vi "Installer.vi"() -> ()   [LabVIEW 2019, in "ByteLVDevEnv.lvlib"]
doc: "VIP Package Installer.\nTakes a txt file with libraries version you want to install and automatically imports them into VIPM and installs them.\nThe txt needs to be formatted this way:\nLibName == 1.1.1.1\nor\n0.0.0.0 > LibName <= 1.1.1.1\nOne library version for line."
uses:
  ByteLVDevEnv.lvlib
  TypeDefs/LibraryVersions.ctl
  TypeDefs/AllLibraries.ctl
  <vilib>/regexp/Match Regular Expression.xnode
  <vilib>/JKI/VIPM API/VIPM API_vipm_api.lvlib
panel:
  in  "Select LabVIEV Version":u16(ring) items=["19.0"]
  out "Status":string
  in  "Exit":bool
  in  "Restart":bool
  out "LOADING":string
  out "Packets file errors":string[](array[string])
  in  "Local VIP Folder":path
  out "VIP files found in local folder":string
  out "Install log":string[](array[string])
  in  "Start":bool
  in  "Packets File Path":path
  # "Development Environment"
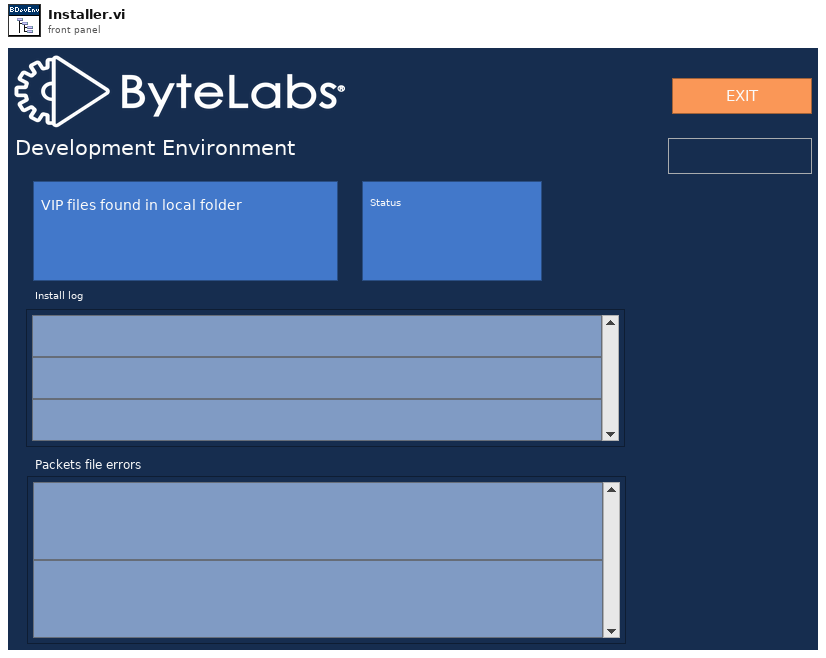
[diagram p1: front panel]
types:
  T1 = typedef "ByteLVDevEnv.lvlib/AllLibraries.ctl" = cluster{"Package Name":string, "Version":string, "Installed":bool, "Path":path}
  T2 = typedef "ByteLVDevEnv.lvlib/LibraryVersions.ctl" = cluster{"Name":string, "Version 1 ":string, "Version 2":string, "Sign 1":string, "Sign 2":string, "Function":string, "V. Install":string}
  T3 = cluster{"LOADING":refnum<vi>, "Local VIP Folder":refnum<vi>, "Packets File Path ":refnum<vi>, "Start":refnum<vi>, "Install log":refnum<vi>, "VIP files found in local folder":refnum<vi>, "Packets file errors":refnum<vi>, "Restart":refnum<vi>, "Exit":refnum<vi>, "Status":refnum<vi>, "Select LabVIEV Version":refnum<vi>}
  T4 = cluster{"Status":string, "Versions":T2[], "All Packages":T1[], "LabView V.":string, "LocalVip":T1[], "Log":string[], "Packets errors":string[]}
  T5 = enum8{"Enabled", "Disabled", "Disabled and Grayed Out"}
  T6 = enum16{"open", "replace", "create", "open or create", "replace or create", "replace or create with confirmation"}
  T7 = cluster{"Packets File Path ":path, "Local VIP Folder":path, "Select LabVIEV Version":u16}
  T8 = typedef "VIPM API_vipm_api.lvlib/LabVIEW Target Info Cluster_vipm_api.ctl" = cluster{"Version":string, "Connection Tested":bool, "Disabled":bool}
  T9 = typedef "LVStringsAndValuesArrayTypeDef_U16.ctl" = cluster{"String":string, "Value":u16}[]
  T10 = typedef "VIPM API_vipm_api.lvlib/Library Contents Cluster_vipm_api.ctl" = cluster{"Package Name":string, "Version":string, "Display Name":string, "Repository Name":string, "Company Name":string, "License Type":string, "Installed":bool, "Deprecated":bool, "Dependency or Conflict Problem":bool, "Downloaded":bool}
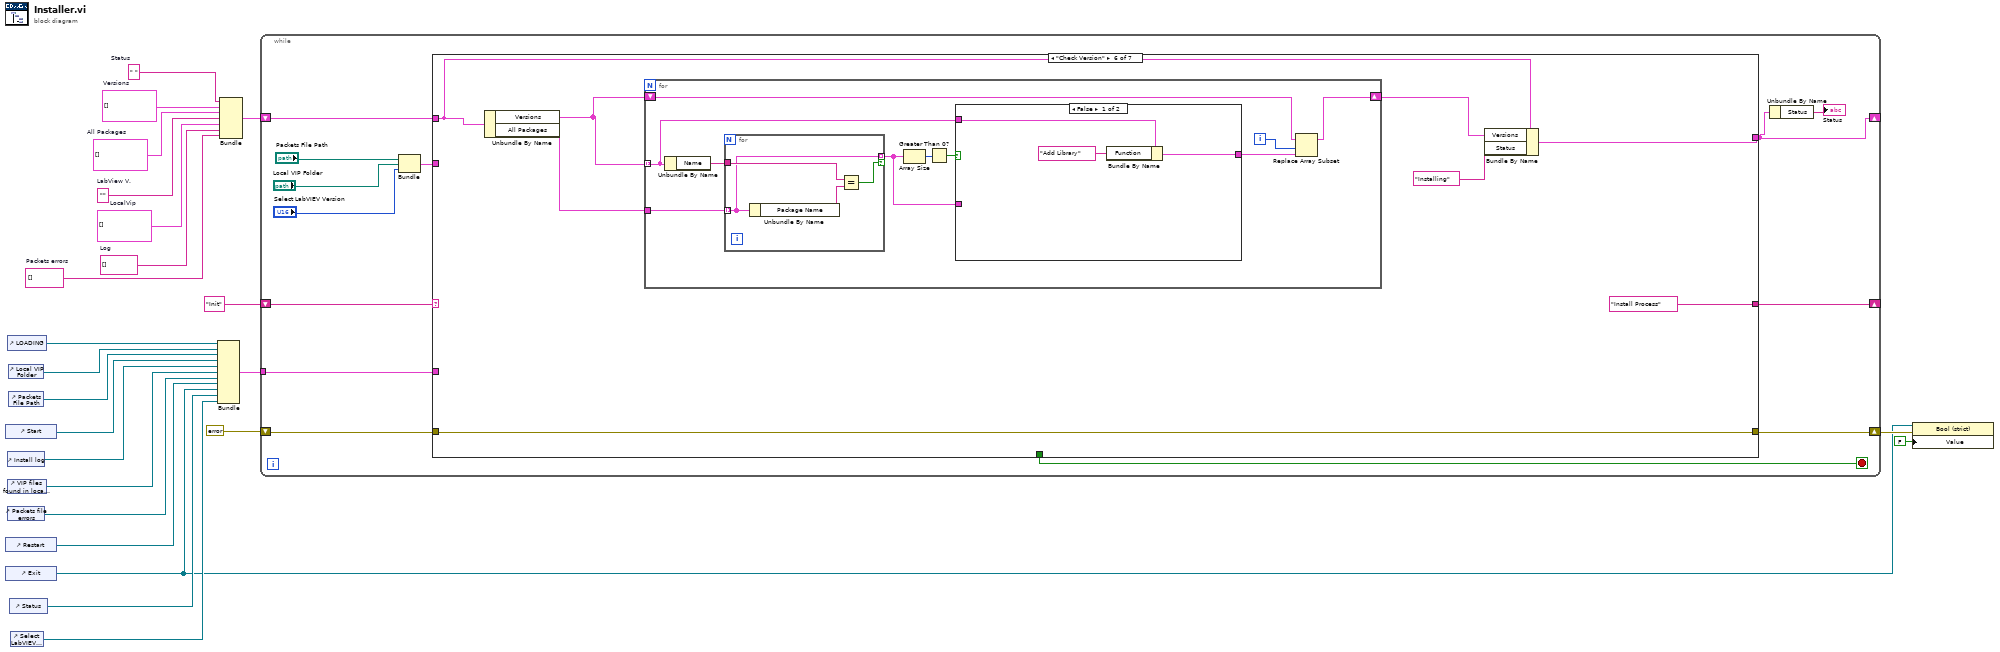
[diagram p0: block diagram]
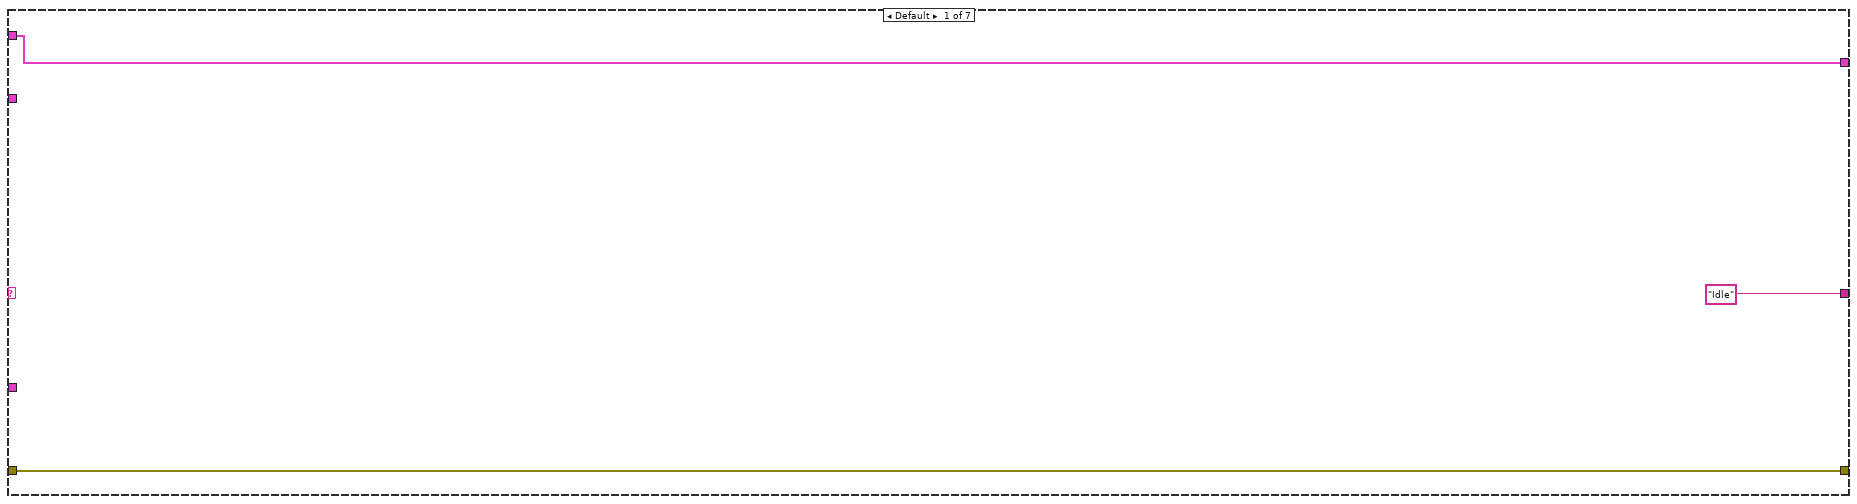
[diagram p2: hidden frame]
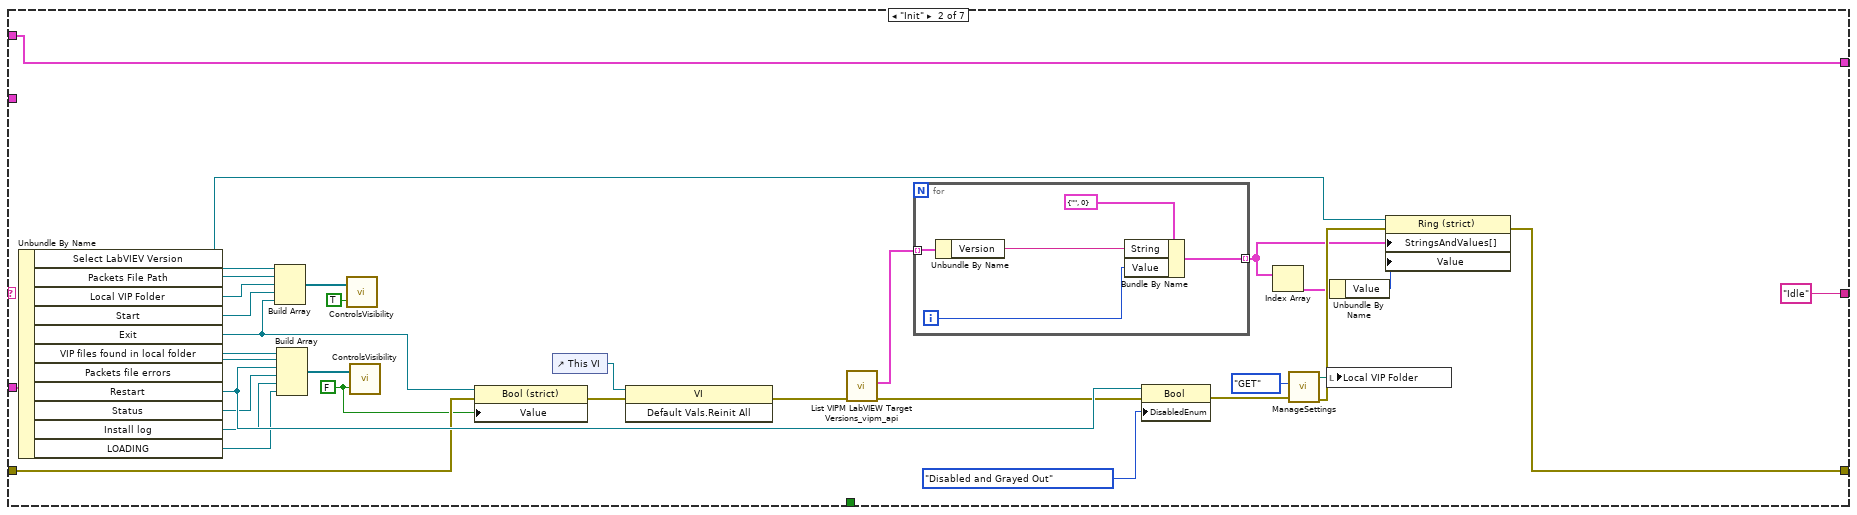
[diagram p3: hidden frame]
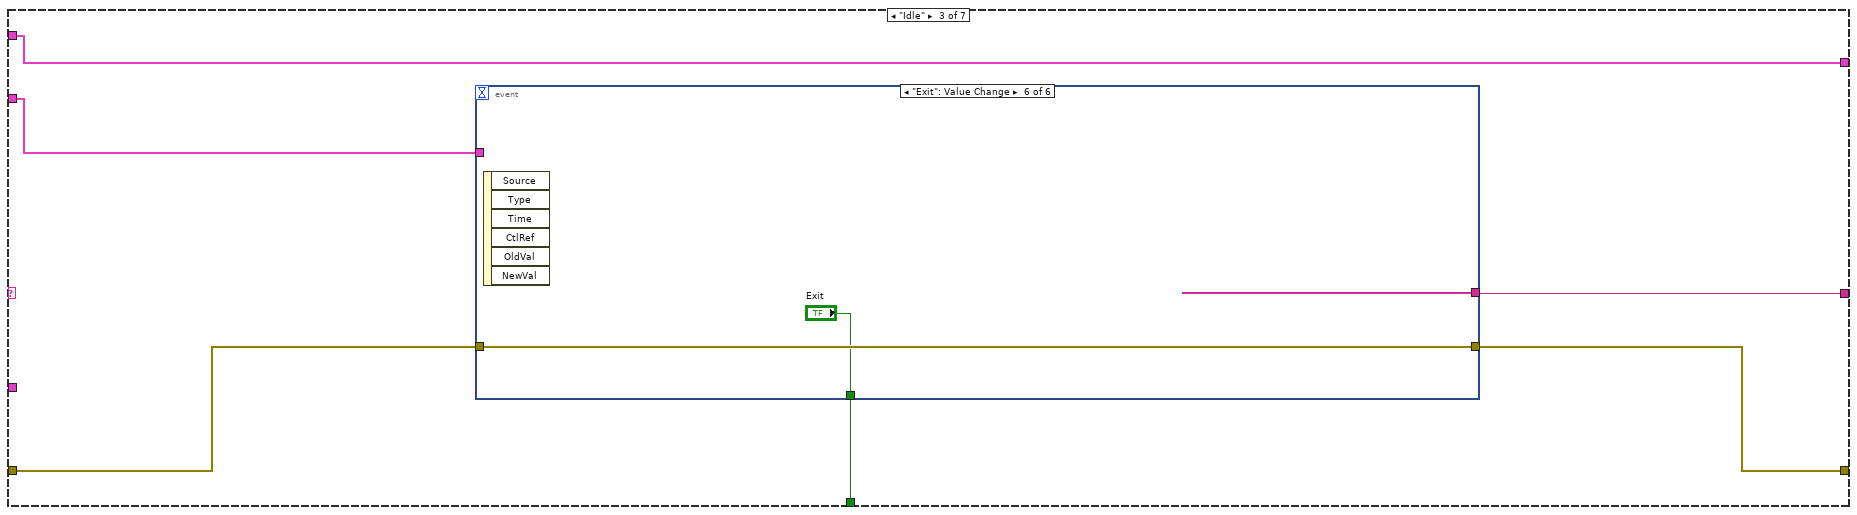
[diagram p4: hidden frame]
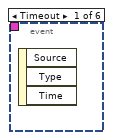
[diagram p5: hidden frame]
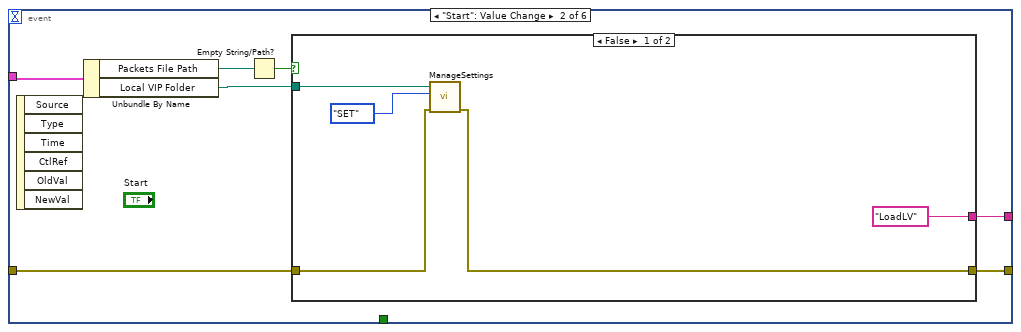
[diagram p6: hidden frame]
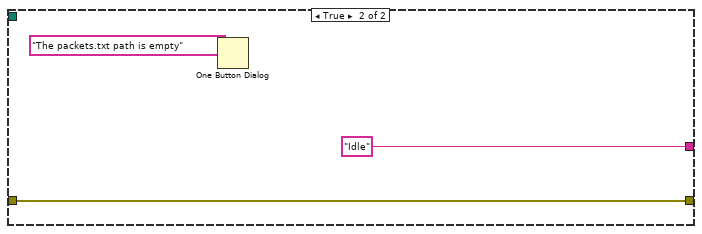
[diagram p7: hidden frame]
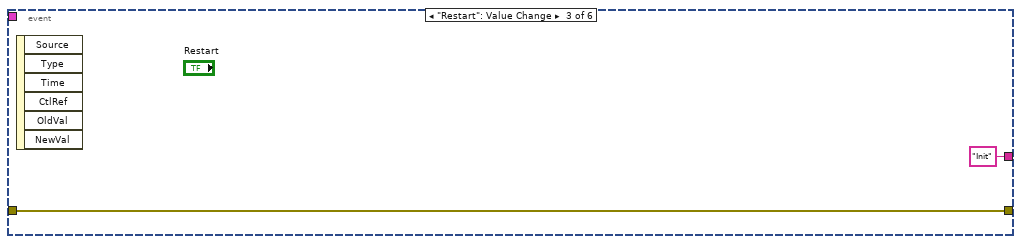
[diagram p8: hidden frame]
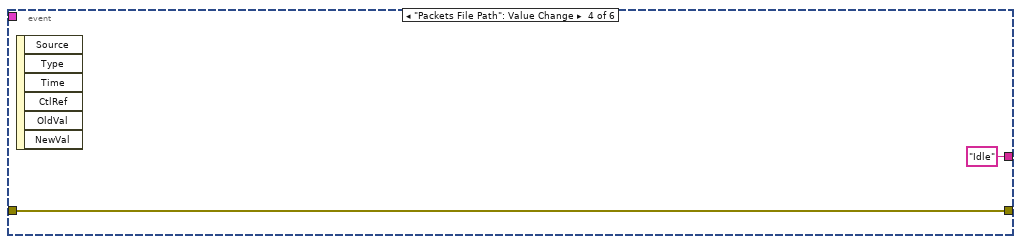
[diagram p9: hidden frame]
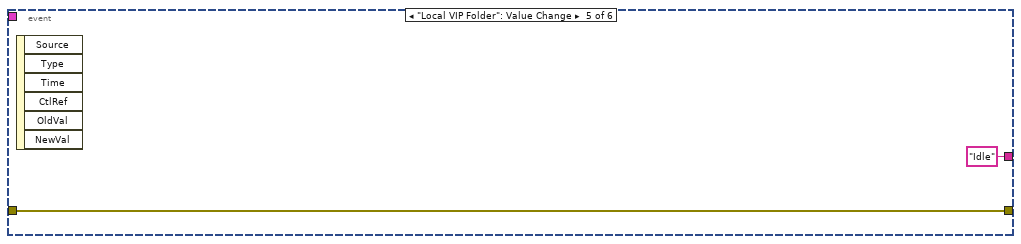
[diagram p10: hidden frame]
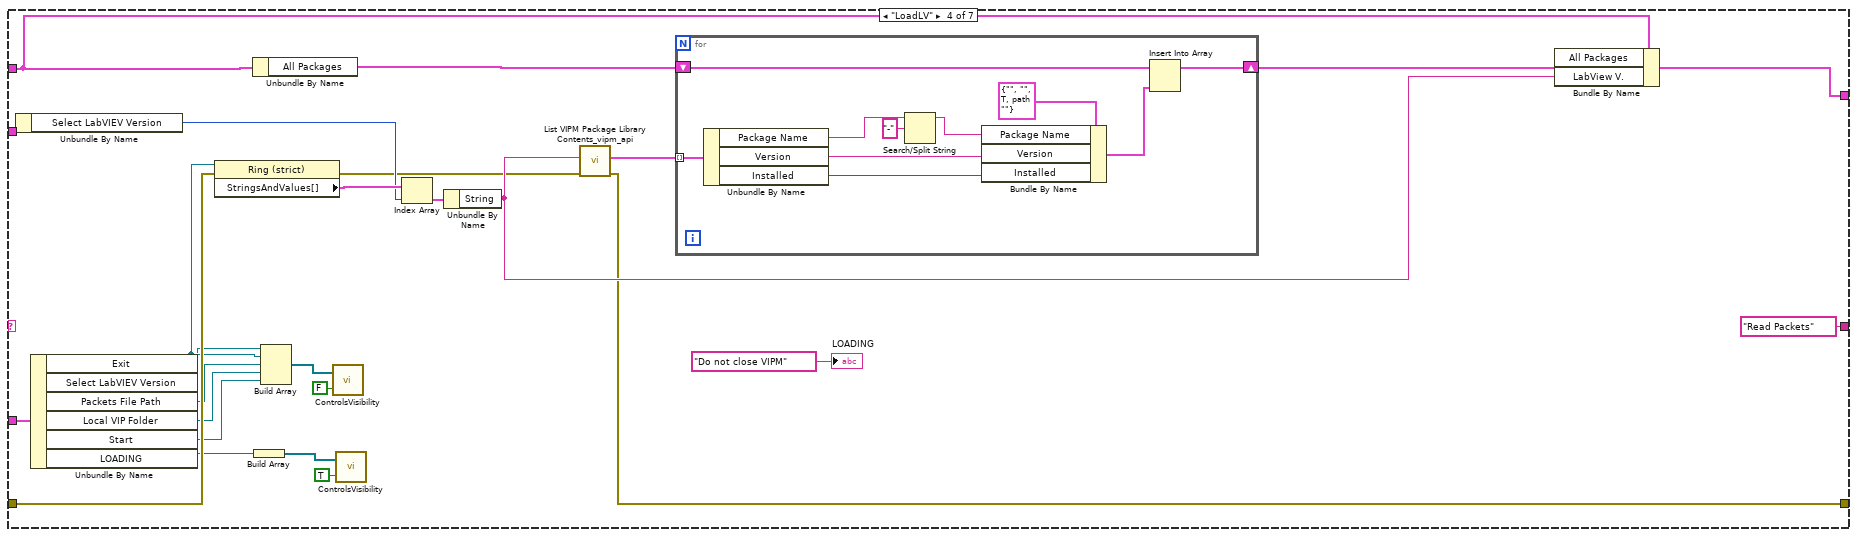
[diagram p11: hidden frame]
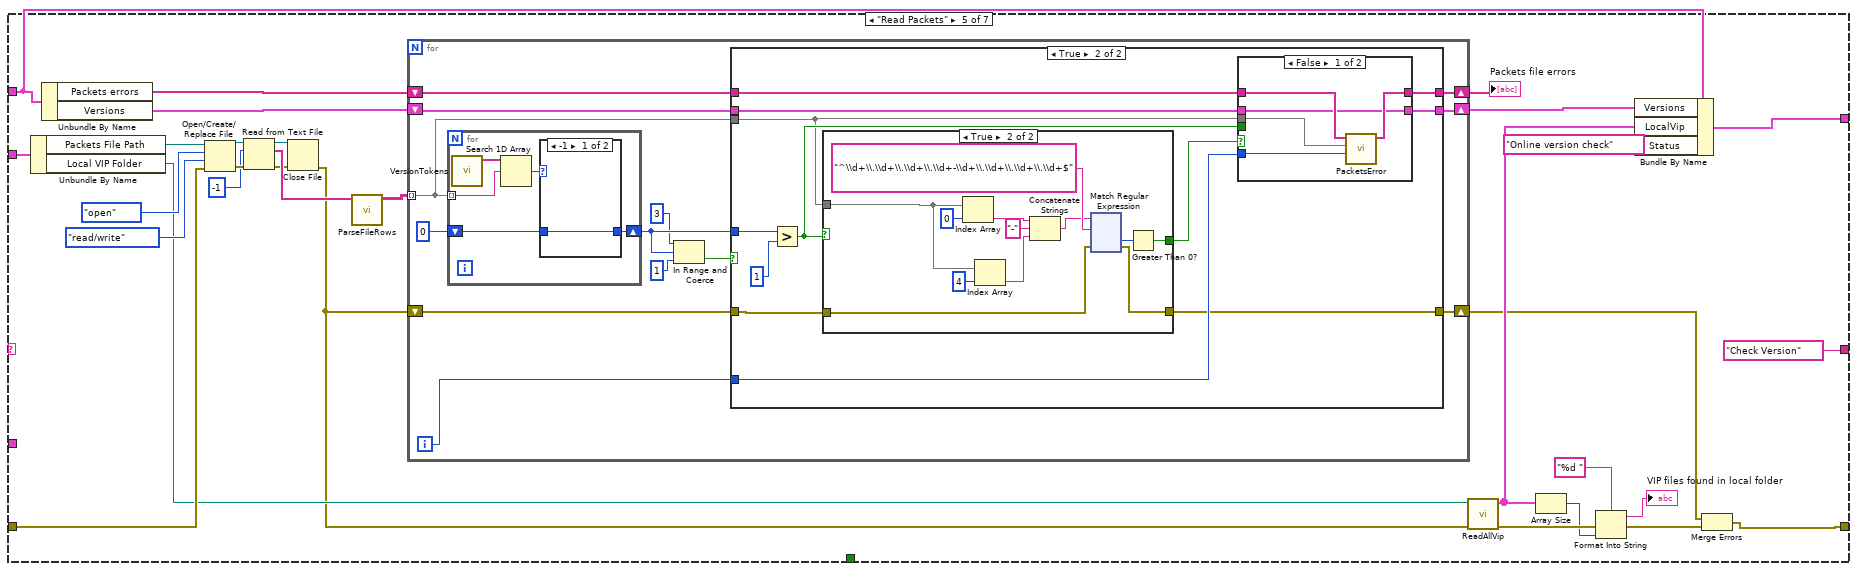
[diagram p12: hidden frame]
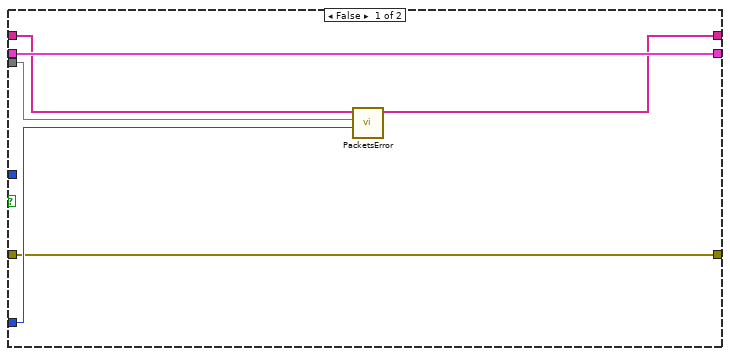
[diagram p13: hidden frame]
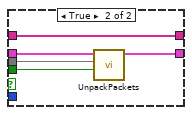
[diagram p14: hidden frame]
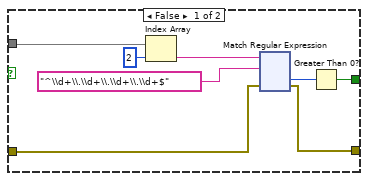
[diagram p15: hidden frame]
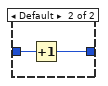
[diagram p16: hidden frame]
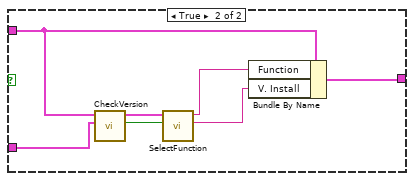
[diagram p17: hidden frame]
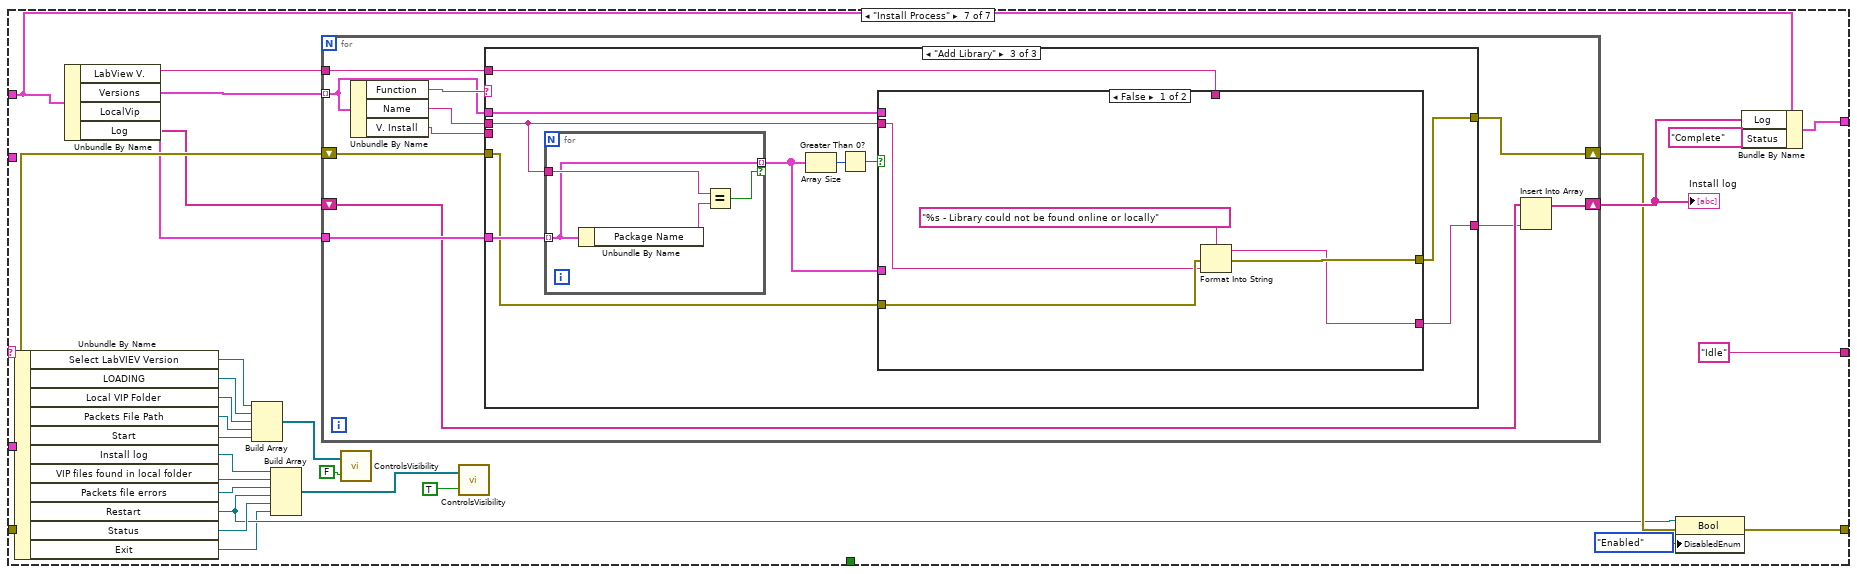
[diagram p18: hidden frame]
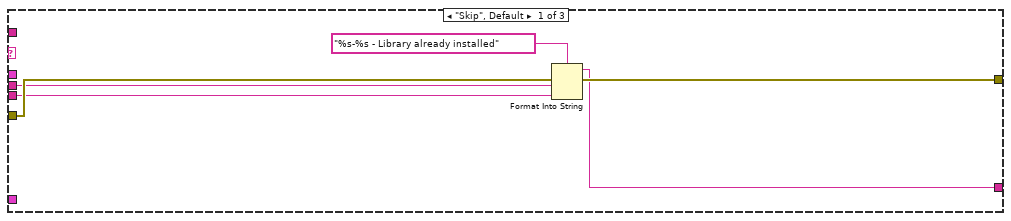
[diagram p19: hidden frame]
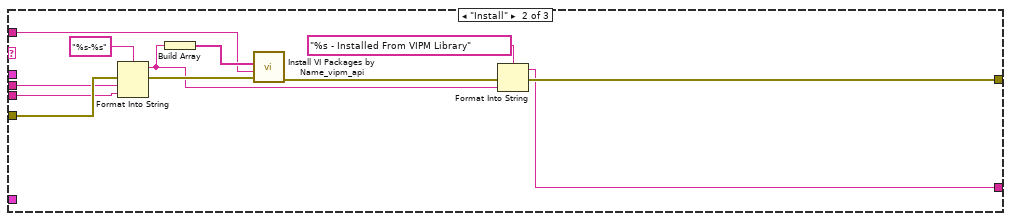
[diagram p20: hidden frame]
diagram:
  w6 = " "  # Status
  w16 = string[] []  # Packets errors
  w17 = string[] []  # Log
  w18 = T1[] []  # LocalVip
  w20 = ""  # LabView V.
  w21 = T1[] []  # All Packages
  w23 = T2[] []  # Versions
  n1 = control-ref of="Start"() -> (w12:refnum<vi>)
  n2 = control-ref of="Restart"() -> (w7:refnum<vi>)
  n3 = control-ref of="Exit"() -> (w1:refnum<vi>)
  n4 = control-ref of="LOADING"() -> (w15:refnum<vi>)
  n5 = control-ref of="Install log"() -> (w11:refnum<vi>)
  n6 = control-ref of="VIP files found in local folder"() -> (w10:refnum<vi>)
  n7 = control-ref of="Packets file errors"() -> (w9:refnum<vi>)
  n8 = control-ref of="Local VIP Folder"() -> (w14:refnum<vi>)
  n9 = control-ref of="Packets File Path"() -> (w13:refnum<vi>)
  n10 = control-ref of="Status"() -> (w5:refnum<vi>)
  n11 = control-ref of="Select LabVIEV Version"() -> (w2:refnum<vi>)
  n12 = Bundle("LOADING"=w15, "Local VIP Folder"=w14, "Packets File Path"=w13, "Start"=w12, "Install log"=w11, "VIP files found in local folder"=w10, "Packets file errors"=w9, "Restart"=w7, "Exit"=w1, "Status"=w5, "Select LabVIEV Version"=w2) -> (w8:T3)  [unwired: 1 in]
  n13 = Bundle("Status"=w6, "Versions"=w23, "All Packages"=w21, "LabView V."=w20, "LocalVip"=w18, "Log"=w17, "Packets errors"=w16) -> (w22:T4)  [unwired: 1 in]
  n14 = while {
    shift-right: [w34] -> _
    shift-left: "Init" -> [w37]
    shift-right: [w27] -> _
    shift-left: w22 -> [w33]
    shift-right: [w32] -> w4
    shift-left: errorcluster {"status"=FALSE, "code"=0, "source"=""} ("error in") -> [w31]
    tunnel: w8 -> [w29]
    stop <- w28 stop-if-true
    n15 = Bundle("Packets File Path"="Packets File Path", "Local VIP Folder"="Local VIP Folder", "Select LabVIEV Version"="Select LabVIEV Version") -> (w35:T7)  [unwired: 1 in]
    n16 = case shown="\"Check Version\"" w37 {
      tunnel: w35 -> [_ _ w82 w125 w173 _ _]
      tunnel: ["Idle" "Idle" w84 "Read Packets" "Check Version" "Install Process" "Idle"] -> w34
      tunnel: w33 -> [w39 w72 w83 w131 w163 w475 w525]
      tunnel: w31 -> [w38 w43 w81 w127 w171 w476 w529]
      tunnel: [w39 w72 w83 w130 w161 w472 w524] -> w27
      tunnel: [w38 w49 w80 w110 w146 w476 w508] -> w32
      tunnel: w29 -> [_ w68 _ w128 _ _ w512]
      tunnel: [_ _ w79 _ _ _ _] -> w28
      frame Default {
      }
      frame "Init" {
        w41 = FALSE ("Visible")
        n17 = Unbundle By Name(w68) -> ("Select LabVIEV Version"=w48:refnum<vi>, "Packets File Path"=w64:refnum<vi>, "Local VIP Folder"=w63:refnum<vi>, "Start"=w62:refnum<vi>, "Exit"=w44:refnum<vi>, "VIP files found in local folder"=w61:refnum<vi>, "Packets file errors"=w60:refnum<vi>, "Restart"=w59:refnum<vi>, "Status"=w58:refnum<vi>, "Install log"=w57:refnum<vi>, "LOADING"=w56:refnum<vi>)
        n18 = Build Array(w48, w64, w63, w62, w44) -> (w54:refnum<vi>[])
        n19 = Build Array(w61, w60, w59, w58, w57, w56) -> (w55:refnum<vi>[])
        n20 = call "ControlsVisibility.vi"("Visible"=TRUE, "Array"=w54) -> ()  [unwired: 2 in]
        n21 = call "ControlsVisibility.vi"("Visible"=w41, "Array"=w55) -> ()  [unwired: 2 in]
        n22 = property class="Bool (strict)"(reference=w44, error in=w43, "Value"=w41) -> (error out=w42:errorcluster)  [unwired: 1 out]
        n23 = control-ref of="This VI"() -> (w70:refnum<vi>)
        n24 = invoke class="VI" method="Default Vals.Reinit All"(reference=w70, error in=w42) -> (error out=w53:errorcluster)  [unwired: 1 in, 2 out]
        n25 = call <vilib>:"List VIPM LabVIEW Target Versions_vipm_api.vi"("error in (no error)"=w53) -> ("error out"=w52:errorcluster, "LabVIEW Target Info"=w51:T8[])  [unwired: 9 in]
        n26 = for {
          tunnel: w51 -> [w77] mode=indexing
          tunnel: [w74] -> w47 mode=indexing
          i -> [w75]
          n27 = Unbundle By Name(w77) -> ("Version"=w76:string)
          n28 = Bundle By Name(cluster=cluster{"String":string, "Value":u16} {"String"="", "Value"=0} ("Cluster"), "String"=w76, "Value"=w75) -> (w74:cluster{"String":string, "Value":u16})
        }
        n29 = property class="Bool"(reference=w59, error in=w52, "DisabledEnum"=T5."Disabled and Grayed Out" ("Disabled")) -> (error out=w66:errorcluster)  [unwired: 1 out]
        n30 = Index Array(array=w47) -> (element=w46:cluster{"String":string, "Value":u16})  [unwired: 1 in]
        n31 = call "ManageSettings.vi"("error in (no error)"=w66, "Mode"=enum16{"GET", "SET"}."GET") -> ("error out"=w50:errorcluster, "File Path Out"=w69:path)  [unwired: 8 in]
        n32 = local write "Local VIP Folder"(w69) -> ()
        n33 = Unbundle By Name(w46) -> ("Value"=w45:u16)
        n34 = property class="Ring (strict)"(reference=w48, error in=w50, "StringsAndValues[]"=w47, "Value"=w45) -> (error out=w49:errorcluster)  [unwired: 1 out]
      }
      frame "Idle" {
        n35 = event shown="[5] \"Exit\": Value Change" {
          selector: _ -> [_ _ _ _ _ _]
          dyn-events: _ -> [_ _ _ _ _ _]
          timeout: _ -> [_ _ _ _ _ _]
          tunnel: [_ w88 "Init" "Idle" "Idle" _] -> w84
          tunnel: w82 -> [_ w91 _ _ _ _]
          tunnel: w81 -> [_ w86 w101 w102 w104 w107]
          tunnel: [_ w85 w101 w102 w104 w107] -> w80
          tunnel: [_ _ _ _ _ "Exit"] -> w79
          event Timeout {
            n36 = event-data() -> ()  [unwired: 1 in, 3 out]
          }
          event "Start": Value Change {
            n37 = event-data() -> ()  [unwired: 1 in, 6 out]
            n38 = Unbundle By Name(w91) -> ("Packets File Path"=w90:path, "Local VIP Folder"=w87:path)
            n39 = Empty String/Path?(string/path=w90) -> (empty?=w89:bool)
            n40 = case shown="False" w89 {
              tunnel: ["LoadLV" "Idle"] -> w88
              tunnel: w87 -> [w95 _]
              tunnel: w86 -> [w93 w98]
              tunnel: [w92 w98] -> w85
              frame False {
                n41 = call "ManageSettings.vi"("error in (no error)"=w93, "Mode"=enum16{"GET", "SET"}."SET", "File Path"=w95) -> ("error out"=w92:errorcluster)  [unwired: 7 in, 1 out]
              }
              frame True {
                n42 = One Button Dialog(message="The packets.txt path is empty") -> ()  [unwired: 1 in, 1 out]
              }
            }
          }
          event "Restart": Value Change {
            n43 = event-data() -> ()  [unwired: 1 in, 6 out]
          }
          event "Packets File Path": Value Change {
            n44 = event-data() -> ()  [unwired: 1 in, 6 out]
          }
          event "Local VIP Folder": Value Change {
            n45 = event-data() -> ()  [unwired: 1 in, 6 out]
          }
          event "Exit": Value Change {
            n46 = event-data() -> ()  [unwired: 1 in, 6 out]
          }
        }
      }
      frame "LoadLV" {
        n47 = Unbundle By Name(w125) -> ("Select LabVIEV Version"=w124:u16)
        n48 = Unbundle By Name(w128) -> ("Exit"=w108:refnum<vi>, "Select LabVIEV Version"=w115:refnum<vi>, "Packets File Path"=w114:refnum<vi>, "Local VIP Folder"=w113:refnum<vi>, "Start"=w112:refnum<vi>, "LOADING"=w111:refnum<vi>)
        n49 = property class="Ring (strict)"(reference=w115, error in=w127) -> (error out=w120:errorcluster, "StringsAndValues[]"=w126:T9)  [unwired: 1 out]
        n50 = Unbundle By Name(w131) -> ("All Packages"=w133:T1[])
        n51 = Build Array(w111) -> (w117:refnum<vi>[])
        n52 = Build Array(w108, w115, w114, w113, w112) -> (w116:refnum<vi>[])
        n53 = call "ControlsVisibility.vi"("Visible"=FALSE, "Array"=w116) -> ()  [unwired: 2 in]
        n54 = call "ControlsVisibility.vi"("Visible"=TRUE, "Array"=w117) -> ()  [unwired: 2 in]
        n55 = Index Array(array=w126, index=w124) -> (element=w123:cluster{"String":string, "Value":u16})
        n56 = Unbundle By Name(w123) -> ("String"=w122:string)
        n57 = call <vilib>:"List VIPM Package Library Contents_vipm_api.vi"("error in (no error)"=w120, "LabVIEW Version"=w122) -> ("error out"=w110:errorcluster, "Library Contents []"=w132:T10[])  [unwired: 7 in, 1 out]
        n58 = for {
          tunnel: w132 -> [w143] mode=indexing
          shift-right: [w136] -> w129
          shift-left: w133 -> [w135]
          n59 = Unbundle By Name(w143) -> ("Package Name"=w141:string, "Version"=w138:string, "Installed"=w137:bool)
          n60 = Search/Split String(string=w141, search string/char (-)="-") -> (substring before match=w139:string)  [unwired: 1 in, 2 out]
          n61 = Bundle By Name(cluster=T1 {"Package Name"="", "Version"="", "Installed"=TRUE, "Path"=path ""}, "Package Name"=w139, "Version"=w138, "Installed"=w137) -> (w134:T1)
          n62 = Insert Into Array(array=w135, new element=w134) -> (w136:T1[])  [unwired: 1 in]
        }
        n63 = Bundle By Name(cluster=w131, "All Packages"=w129, "LabView V."=w122) -> (w130:T4)
        "LOADING" <- "Do not close VIPM" ("LOADING")
      }
      frame "Read Packets" {
        n64 = Unbundle By Name(w173) -> ("Packets File Path"=w172:path, "Local VIP Folder"=w159:path)
        n65 = Unbundle By Name(w163) -> ("Packets errors"=w153:string[], "Versions"=w164:T2[])
        n66 = Open/Create/Replace File(file path (use dialog)=w172, error in=w171, operation (0:open)=T6."open", access (0:read/write)=enum16{"read/write", "read-only", "write-only"}."read/write") -> (refnum out=w168:refnum<file>, error out=w167:errorcluster)  [unwired: 2 in, 1 out]
        n67 = Read from Text File(file (use dialog)=w168, count=-1, error in=w167) -> (refnum out=w149:refnum<file>, text=w166:string[], error out=w150:errorcluster)  [unwired: 1 in, 1 out]
        n68 = Close File(refnum=w149, error in=w150) -> (error out=w148:errorcluster)  [unwired: 1 out]
        n69 = call "ParseFileRows.vi"("file rows"=w166) -> ("packages"=w165:string[][])  [unwired: 10 in]
        n70 = for {
          tunnel: w165 -> [w183] mode=indexing
          shift-right: [w185] -> w162
          shift-left: w164 -> [w186]
          shift-right: [w177] -> w152
          shift-left: w153 -> [w178]
          shift-right: [w174] -> w145
          shift-left: w148 -> [w175]
          i -> [w176]
          n71 = for {
            tunnel: w183 -> [w464] mode=indexing
            shift-right: [w466] -> w182
            shift-left: 0 -> [w467]
            n72 = call "VersionTokens.vi"() -> ("Array"=w465:string[])  [unwired: 11 in]
            n73 = Search 1D Array(1D array=w465, element=w464) -> (index of element=w463:i32)  [unwired: 1 in]
            n74 = case shown="-1" w463 {
              tunnel: w467 -> [w468 w470]
              tunnel: [w468 w469] -> w466
              frame -1 {
              }
              frame Default {
                n75 = Increment(x=w470) -> (x+1=w469:i32)
              }
            }
          }
          n76 = In Range and Coerce(upper limit=3, x=w182, lower limit=1) -> (In Range?=w179:bool)  [unwired: 1 out]
          n77 = case shown="True" w179 {
            tunnel: w186 -> [w192 w204]
            tunnel: [w192 w203] -> w185
            tunnel: w183 -> [w191 w199]
            tunnel: w182 -> [_ w201]
            tunnel: w178 -> [w190 w198]
            tunnel: [w189 w197] -> w177
            tunnel: w176 -> [w188 w196]
            tunnel: w175 -> [w187 w194]
            tunnel: [w187 w193] -> w174
            frame False {
              n78 = call "PacketsError.vi"("Index"=w188, "Libraries"=w191, "Packets errors in"=w190) -> ("Packets errors out"=w189:string[])  [unwired: 8 in]
            }
            frame True {
              n79 = Greater?(x=w201, y=1) -> (0:w200:bool)
              n80 = case shown="True" w200 {
                tunnel: w199 -> [w222 w344]
                tunnel: [w218 w343] -> w195
                tunnel: w194 -> [w216 w338]
                tunnel: [w215 w337] -> w193
                frame False {
                  n81 = Index Array(array=w222, index=2) -> (element=w220:string)
                  n82 = xnode "Match Regular Expression"("input string"=w220, "regular expression"="^\\d+\\.\\d+\\.\\d+\\.\\d+$", "error in"=w216) -> ("offset past match"=w217:i32, "error out"=w215:errorcluster)  [unwired: 3 in, 3 out]
                  n83 = Greater Than 0?(x=w217) -> (x > 0?=w218:bool)
                }
                frame True {
                  n84 = Index Array(array=w344, index=0) -> (element=w342:string)
                  n85 = Index Array(array=w344, index=4) -> (element=w341:string)
                  n86 = Concatenate Strings(w342, "-" ("string"), w341) -> (w339:string)
                  n87 = xnode "Match Regular Expression"("input string"=w339, "regular expression"="^\\d+\\.\\d+\\.\\d+\\.\\d+-\\d+\\.\\d+\\.\\d+\\.\\d+$", "error in"=w338) -> ("offset past match"=w346:i32, "error out"=w337:errorcluster)  [unwired: 3 in, 3 out]
                  n88 = Greater Than 0?(x=w346) -> (x > 0?=w343:bool)
                }
              }
              n89 = case shown="False" w195 {
                tunnel: w204 -> [w206 w214]
                tunnel: [w206 w213] -> w203
                tunnel: w200 -> [_ w212]
                tunnel: w199 -> [w205 w211]
                tunnel: w198 -> [w208 w210]
                tunnel: [w207 w210] -> w197
                tunnel: w196 -> [w209 _]
                frame False {
                  n90 = call "PacketsError.vi"("Index"=w209, "Libraries"=w205, "Packets errors in"=w208) -> ("Packets errors out"=w207:string[])  [unwired: 8 in]
                }
                frame True {
                  n91 = call "UnpackPackets.vi"("Type"=w212, "Libraries"=w211, "Versions in"=w214) -> ("Versions out"=w213:T2[])  [unwired: 8 in]
                }
              }
            }
          }
        }
        "Packets file errors" <- w152
        n92 = call "ReadAllVip.vi"("error in (no error)"=w148, "Cartella VIP locale"=w159) -> ("error out"=w157:errorcluster, "LocalVip"=w158:T1[])  [unwired: 8 in]
        n93 = Array Size(array=w158) -> (size(s)=w156:i32)
        n94 = Format Into String(format string="%d ", error in=w157, w156) -> (resulting string=→"VIP files found in local folder":string, error out=w147:errorcluster)  [unwired: 1 in]
        n95 = Bundle By Name(cluster=w163, "Versions"=w162, "LocalVip"=w158, "Status"="Online version check") -> (w161:T4)
        n96 = Merge Errors(w145, w147) -> (w146:errorcluster)
      }
      frame "Check Version" {
        n97 = Unbundle By Name(w475) -> ("Versions"=w474:T2[], "All Packages"=w477:T1[])
        n98 = for {
          tunnel: w474 -> [w483] mode=indexing
          tunnel: w477 -> [w488]
          shift-right: [w479] -> w473
          shift-left: w474 -> [w480]
          i -> [w482]
          n99 = Unbundle By Name(w483) -> ("Name"=w487:string)
          n100 = for {
            tunnel: w488 -> [w500] mode=indexing
            tunnel: w487 -> [w501]
            tunnel: [w500] -> w484 mode=indexing if=w499
            n101 = Unbundle By Name(w500) -> ("Package Name"=w502:string)
            n102 = Equal?(x=w501, y=w502) -> (x = y?=w499:bool)
          }
          n103 = Array Size(array=w484) -> (size(s)=w486:i32)
          n104 = Greater Than 0?(x=w486) -> (x > 0?=w485:bool)
          n105 = case shown="False" w485 {
            tunnel: w484 -> [_ w497]
            tunnel: w483 -> [w491 w496]
            tunnel: [w489 w498] -> w481
            frame False {
              n106 = Bundle By Name(cluster=w491, "Function"="Add Library") -> (w489:T2)
            }
            frame True {
              n107 = call "CheckVersion.vi"("packages"=w497, "versions"=w496) -> ("found"=w494:bool, "package version"=w495:T1)  [unwired: 8 in]
              n108 = call "SelectFunction.vi"("Found?"=w494, "Library"=w495) -> ("Version"=w492:string, "Function"=w493:string)  [unwired: 8 in]
              n109 = Bundle By Name(cluster=w496, "Function"=w493, "V. Install"=w492) -> (w498:T2)
            }
          }
          n110 = Replace Array Subset(array=w480, new element=w481, index=w482) -> (w479:T2[])
        }
        n111 = Bundle By Name(cluster=w475, "Versions"=w473, "Status"="Installing") -> (w472:T4)
      }
      frame "Install Process" {
        n112 = Unbundle By Name(w512) -> ("Select LabVIEV Version"=w504:refnum<vi>, "LOADING"=w505:refnum<vi>, "Local VIP Folder"=w522:refnum<vi>, "Packets File Path"=w521:refnum<vi>, "Start"=w520:refnum<vi>, "Install log"=w517:refnum<vi>, "VIP files found in local folder"=w516:refnum<vi>, "Packets file errors"=w515:refnum<vi>, "Restart"=w507:refnum<vi>, "Status"=w510:refnum<vi>, "Exit"=w503:refnum<vi>)
        n113 = Unbundle By Name(w525) -> ("LabView V."=w528:string, "Versions"=w530:T2[], "LocalVip"=w527:T1[], "Log"=w526:string[])
        n114 = Build Array(w504, w505, w522, w521, w520) -> (w514:refnum<vi>[])
        n115 = Build Array(w517, w516, w515, w507, w510, w503) -> (w513:refnum<vi>[])
        n116 = for {
          tunnel: w530 -> [w535] mode=indexing
          shift-right: [w537] -> w509
          shift-left: w529 -> [w541]
          tunnel: w528 -> [w538]
          tunnel: w527 -> [w536]
          shift-right: [w532] -> w523
          shift-left: w526 -> [w534]
          n117 = Unbundle By Name(w535) -> ("Function"=w542:string, "Name"=w540:string, "V. Install"=w539:string)
          n118 = case shown="\"Add Library\"" w542 {
            tunnel: w541 -> [w548 w559 w565]
            tunnel: w540 -> [w544 w557 w561]
            tunnel: w539 -> [w543 w556 _]
            tunnel: w538 -> [_ w554 w563]
            tunnel: [w547 w550 w564] -> w537
            tunnel: w536 -> [_ _ w567]
            tunnel: w535 -> [_ _ w566]
            tunnel: [w545 w549 w562] -> w533
            frame "Skip", Default {
              n119 = Format Into String(format string="%s-%s - Library already installed", error in=w548, w544, w543) -> (resulting string=w545:string, error out=w547:errorcluster)  [unwired: 1 in]
            }
            frame "Install" {
              n120 = Format Into String(format string="%s-%s", error in=w559, w557, w556) -> (resulting string=w551:string, error out=w558:errorcluster)  [unwired: 1 in]
              n121 = Build Array(w551) -> (w555:string[])
              n122 = call <vilib>:"Install VI Packages by Name_vipm_api.vi"("error in (no error)"=w558, "LabVIEW Version"=w554, "Package Names to Install []"=w555) -> ("error out"=w552:errorcluster)  [unwired: 8 in]
              n123 = Format Into String(format string="%s - Installed From VIPM Library", error in=w552, w551) -> (resulting string=w549:string, error out=w550:errorcluster)  [unwired: 1 in]
            }
            frame "Add Library" {
              n124 = for {
                tunnel: w567 -> [w604] mode=indexing
                tunnel: w561 -> [w605]
                tunnel: [w604] -> w568 mode=indexing if=w603
                n125 = Unbundle By Name(w604) -> ("Package Name"=w606:string)
                n126 = Equal?(x=w605, y=w606) -> (x = y?=w603:bool)
              }
              n127 = Array Size(array=w568) -> (size(s)=w570:i32)
              n128 = Greater Than 0?(x=w570) -> (x > 0?=w569:bool)
              n129 = case shown="False" w569 {
                tunnel: w568 -> [_ w584]
                tunnel: w566 -> [_ w583]
                tunnel: w565 -> [w575 w580]
                tunnel: [w574 w579] -> w564
                tunnel: w563 -> [_ w578]
                tunnel: [w572 w577] -> w562
                tunnel: w561 -> [w571 w576]
                frame False {
                  n130 = Format Into String(format string="%s - Library could not be found online or locally", error in=w575, w571) -> (resulting string=w572:string, error out=w574:errorcluster)  [unwired: 1 in]
                }
                frame True {
                  n131 = call "CheckVersion.vi"("packages"=w584, "versions"=w583) -> ("found"=w582:bool, "package version"=w581:T1)  [unwired: 8 in]
                  n132 = case shown="True" w582 {
                    tunnel: w581 -> [_ w602]
                    tunnel: w580 -> [w588 w597]
                    tunnel: [w587 w594] -> w579
                    tunnel: w578 -> [_ w596]
                    tunnel: [w586 w590] -> w577
                    tunnel: w576 -> [w585 _]
                    frame False {
                      n133 = Format Into String(format string="%s - Version of Library could not be found online or locally", error in=w588, w585) -> (resulting string=w586:string, error out=w587:errorcluster)  [unwired: 1 in]
                    }
                    frame True {
                      n134 = Unbundle By Name(w602) -> ("Package Name"=w592:string, "Version"=w591:string, "Path"=w601:path)
                      n135 = Build Array(w601) -> (w600:path[])
                      n136 = call <vilib>:"Add VI Packages to VIPM Package Library_vipm_api.vi"("error in (no error)"=w597, "Packages to add to VIPM Library (vipc,vip,ogp)"=w600) -> ("error out"=w599:errorcluster, "Package Names Added"=w598:string[])  [unwired: 8 in]
                      n137 = call <vilib>:"Install VI Packages by Name_vipm_api.vi"("error in (no error)"=w599, "LabVIEW Version"=w596, "Package Names to Install []"=w598) -> ("error out"=w595:errorcluster)  [unwired: 8 in]
                      n138 = Format Into String(format string="%s-%s - Installed from local folder", error in=w595, w592, w591) -> (resulting string=w590:string, error out=w594:errorcluster)  [unwired: 1 in]
                    }
                  }
                }
              }
            }
          }
          n139 = Insert Into Array(array=w534, new element=w533) -> (w532:string[])  [unwired: 1 in]
        }
        "Install log" <- w523
        n140 = call "ControlsVisibility.vi"("Visible"=FALSE, "Array"=w514) -> ()  [unwired: 2 in]
        n141 = call "ControlsVisibility.vi"("Visible"=TRUE, "Array"=w513) -> ()  [unwired: 2 in]
        n142 = property class="Bool"(reference=w507, error in=w509, "DisabledEnum"=T5."Enabled" ("Disabled")) -> (error out=w508:errorcluster)  [unwired: 1 out]
        n143 = Bundle By Name(cluster=w525, "Log"=w523, "Status"="Complete") -> (w524:T4)
      }
    }
    n144 = Unbundle By Name(w27) -> ("Status"=→"Status":string)
  }
  n145 = property class="Bool (strict)"(reference=w1, error in=w4, "Value"=FALSE) -> ()  [unwired: 2 out]
